vi "Comparator_IDs_ForExchange-1.vi"(1 "Min ID Iter#1":u16, 2 "Initial ID":u16, 3 "Biggest ID (init)":u16, 4 "Current ID":u16) -> (0 "ID = old ID":bool)   [LabVIEW 2017]
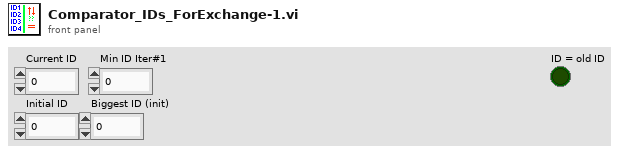
[diagram p1: front panel]
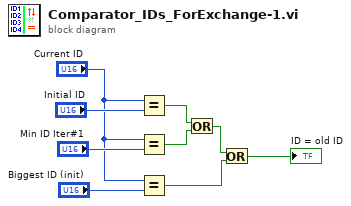
[diagram p0: block diagram]
diagram:
  n1 = Equal?(x="Current ID", y="Initial ID") -> (x = y?=w5:bool)
  n2 = Equal?(x="Current ID", y="Min ID Iter#1") -> (x = y?=w4:bool)
  n3 = Equal?(x="Current ID", y="Biggest ID (init)") -> (x = y?=w2:bool)
  n4 = Or(x=w5, y=w4) -> (x .or. y?=w3:bool)
  n5 = Or(x=w3, y=w2) -> (x .or. y?=→"ID = old ID":bool)
